vi "CorrectDistance.vi"(3 "CenterPoint":dbl=1.0 format="%#_13g", 5 "Distance":dbl=26.11869999999999 format="%#_13g") -> (19 "In Range?":bool, 21 "Right Motor":dbl=1.0 format="%#_13g", 22 "Left Motor":dbl=1.0 format="%#_13g")   [LabVIEW 2016]
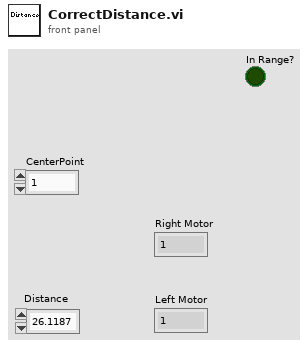
[diagram p1: front panel]
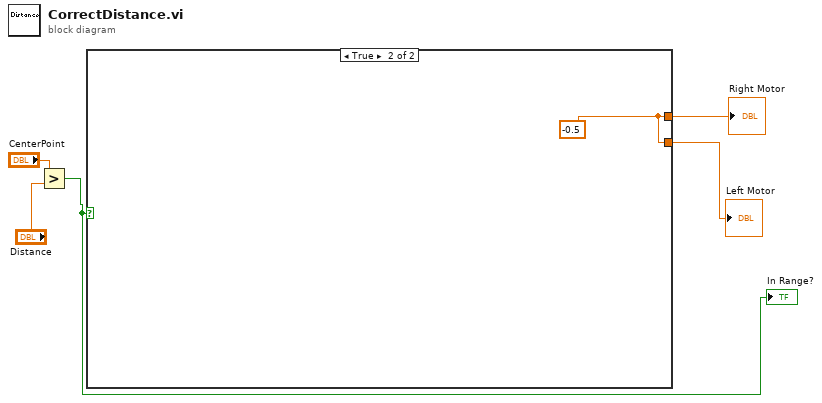
[diagram p0: block diagram]
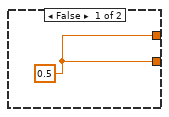
[diagram p2: hidden frame]
diagram:
  n1 = Greater?(x="CenterPoint", y="Distance") -> (0:w1:bool)
  "In Range?" <- w1
  n2 = case shown="True" w1 {
    tunnel: [w6 w7] -> w3
    tunnel: [w6 w7] -> w2
    frame False {
      w6 = 0.5
    }
    frame True {
      w7 = -0.5
    }
  }
  "Right Motor" <- w3
  "Left Motor" <- w2
